vi "Get Resistance.vi"(8 "error in (no error)":errorcluster, 11 "Agilent 3458A in":refnum<class "Agilent 3458A.lvclass">) -> (0 "error out":errorcluster, 2 "Resistance":dbl, 3 "Agilent 3458A out":refnum<class "Agilent 3458A.lvclass">)   [LabVIEW 2011, in "Agilent 3458A.lvclass"]
uses:
  Agilent 3458A.lvclass
  <instrlib>/Agilent 3458/Public/Data/Read Measurement(Single Point).vi
  <instrlib>/Agilent 3458/Agilent 3458.lvlib
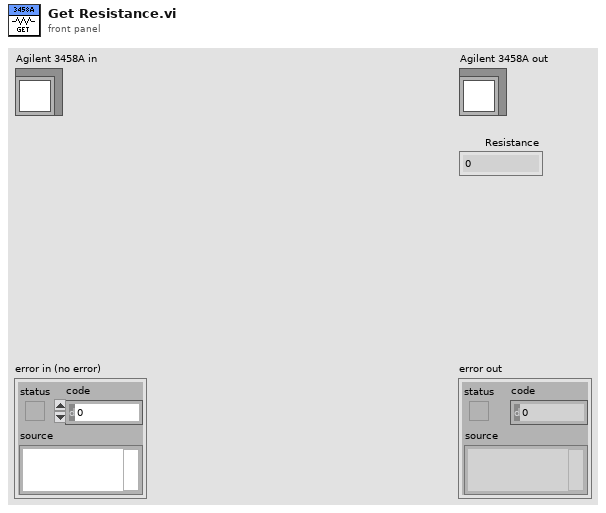
[diagram p1: front panel]
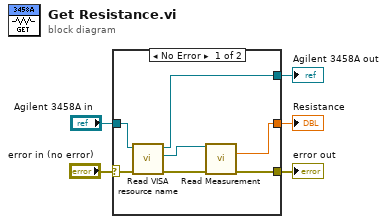
[diagram p0: block diagram]
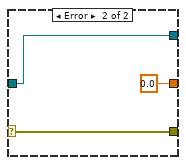
[diagram p2: hidden frame]
diagram:
  n1 = case shown="No Error" "error in (no error)" {
    selector: "error in (no error)" -> [w11 w15]
    tunnel: [w6 w15] -> w4
    tunnel: [w10 w14] -> w2
    tunnel: "Agilent 3458A in" -> [w12 w14]
    tunnel: [w8 0.0 ("Measurement")] -> w1
    frame No Error {
      n2 = call-dynamic "Read VISA resource name.vi"("error in (no error)"=w11, "Multimeter in"=w12) -> ("error out"=w7:errorcluster, "VISA resource name"=w9:refnum<visa-resource-name>, "Multimeter out"=w10:refnum<class "Agilent 3458A.lvclass">)  [unwired: 7 in]
      n3 = call-poly <instrlib>:"Read Measurement.vi"("VISA resource name"=w9, "error in (no error)"=w7) -> ("Measurement"=w8:dbl, "error out"=w6:errorcluster)  [unwired: 11 in, 1 out]
    }
    frame Error {
    }
  }
  "error out" <- w4
  "Agilent 3458A out" <- w2
  "Resistance" <- w1
